vi "Set JSON Data.vi"(7 "VI Reference":refnum<vi>, 8 "error in (no error)":errorcluster, 10 "Value":string, 11 "Numeric In":refnum<class "Numeric.lvclass">) -> (0 "error out":errorcluster, 3 "Numeric Out":refnum<class "Numeric.lvclass">)   [LabVIEW 2017, in "Front Panel Publisher.lvlib" / "Numeric.lvclass"]
uses:
  Numeric.lvclass
  Object_class/Object.lvclass
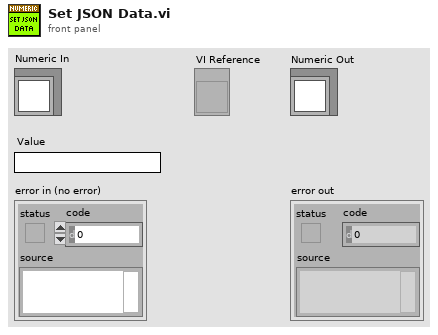
[diagram p1: front panel]
types:
  T1 = typedef "Front Panel Publisher.lvlib/Object.lvclass/Attributes.ctl" = cluster{"UID":i32, "Type":string, "Starting Location":T2, "Reference":refnum<vi>, "Cluster Component":bool, "Starting Rect Position":cluster{"Left":i16, "Top":i16}, "Owning Pane":refnum<vi>, "Master Total Rect Delta":T3}
  T2 = typedef "Front Panel Publisher.lvlib/Object.lvclass/Coordinates.ctl" = cluster{"Left":i32, "Top":i32, "Height":u32, "Width":u32}
  T3 = typedef "LVRectTypeDef.ctl" = cluster{"Left":i16, "Top":i16, "Right":i16, "Bottom":i16}
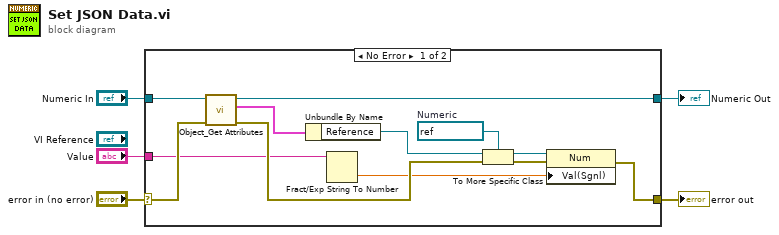
[diagram p0: block diagram]
diagram:
  n1 = case shown="No Error" "error in (no error)" {
    selector: "error in (no error)" -> [w17 w19]
    tunnel: [w16 w19] -> w4
    tunnel: [w11 w18] -> w2
    tunnel: "Numeric In" -> [w12 w18]
    tunnel: "Value" -> [w10 _]
    frame No Error {
      w6 = refnum<vi> refnum  # Numeric
      n2 = call "Object_Get Attributes.vi"("error in (no error)"=w17, "Object In"=w12) -> ("error out"=w15:errorcluster, "Object Attributes"=w13:T1, "Object Out"=w11:refnum<class "Numeric.lvclass">)  [unwired: 7 in]
      n3 = Unbundle By Name(w13) -> ("Reference"=w9:refnum<vi>)
      n4 = Fract/Exp String To Number(string=w10) -> (number=w8:dbl)  [unwired: 3 in, 1 out]
      n5 = To More Specific Class(target class=w6, reference=w9, error in=w15) -> (specific class reference=w7:refnum<vi>, error out=w14:errorcluster)
      n6 = property class="Num"(reference=w7, error in=w14, "Val(Sgnl)"=w8) -> (error out=w16:errorcluster)  [unwired: 1 out]
    }
    frame Error {
    }
  }
  "error out" <- w4
  "Numeric Out" <- w2
